vi "Write connection.vi"(8 "error in (no error)":errorcluster, 10 "connection":refnum<k24>, 11 "DbConnection in":refnum<class "DbConnection.lvclass">) -> (0 "error out":errorcluster, 3 "DbConnection out":refnum<class "DbConnection.lvclass">)   [LabVIEW 2020, in "ORM.lvlib" / "DbConnection.lvclass"]
uses:
  DbConnection.lvclass
  System.Data
  DbConnection.lvclass/DbConnection.ctl
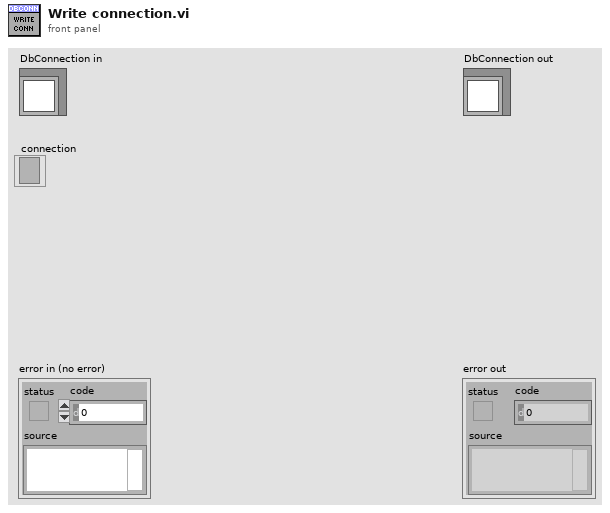
[diagram p1: front panel]
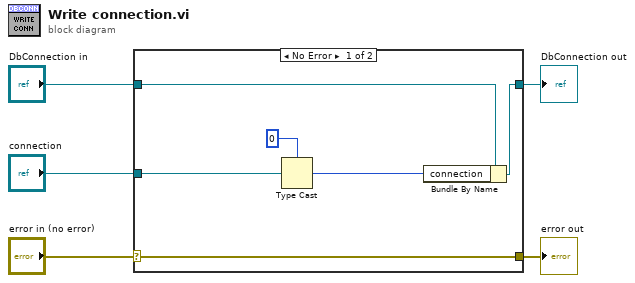
[diagram p0: block diagram]
diagram:
  n1 = case shown="No Error" "error in (no error)" {
    selector: "error in (no error)" -> [w11 w12]
    tunnel: [w11 w12] -> w4
    tunnel: [w9 w13] -> w2
    tunnel: "DbConnection in" -> [w10 w13]
    tunnel: "connection" -> [w8 _]
    frame No Error {
      n2 = Type Cast(type=u64 0 ("connection"), x=w8) -> (*(type *) &x=w6:u64)
      n3 = Bundle By Name(cluster=w10, "connection"=w6) -> (w9:refnum<class "DbConnection.lvclass">)
    }
    frame Error {
    }
  }
  "error out" <- w4
  "DbConnection out" <- w2
